vi "SUB-BLE Rx data Classify.vi"() -> (0 "data out":u8[](array[numeric]) format="%2x", 1 "Rx-set":bool=TRUE, 2 "Rx-mon":bool=TRUE)   [LabVIEW 2015]
doc: "Use this template to create an application that executes repeatedly until you click the Stop button. This template polls the state of the Stop button and does not use events. Use the Top-Level Application template (not available in the Base package) to create a single-loop application with event handling."
uses:
  Global 1.vi
panel:
  out "BLE Packet (buf)":u8[](array[numeric])
  out "BLE Packet (data)":u8[](array[numeric])
  out "BLE Packet":bool=TRUE
  # "BLE 수신 데이터를 분류: Monitoring/Setting data"
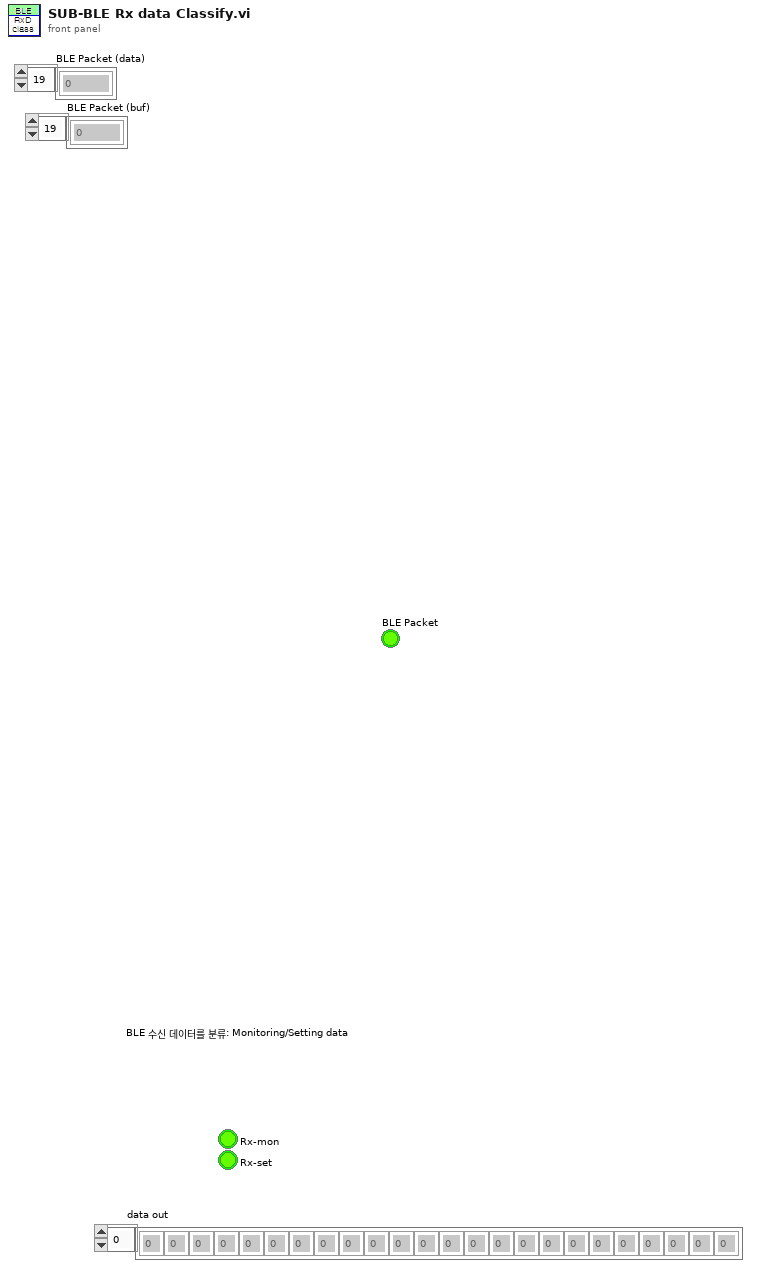
[diagram p1: front panel]
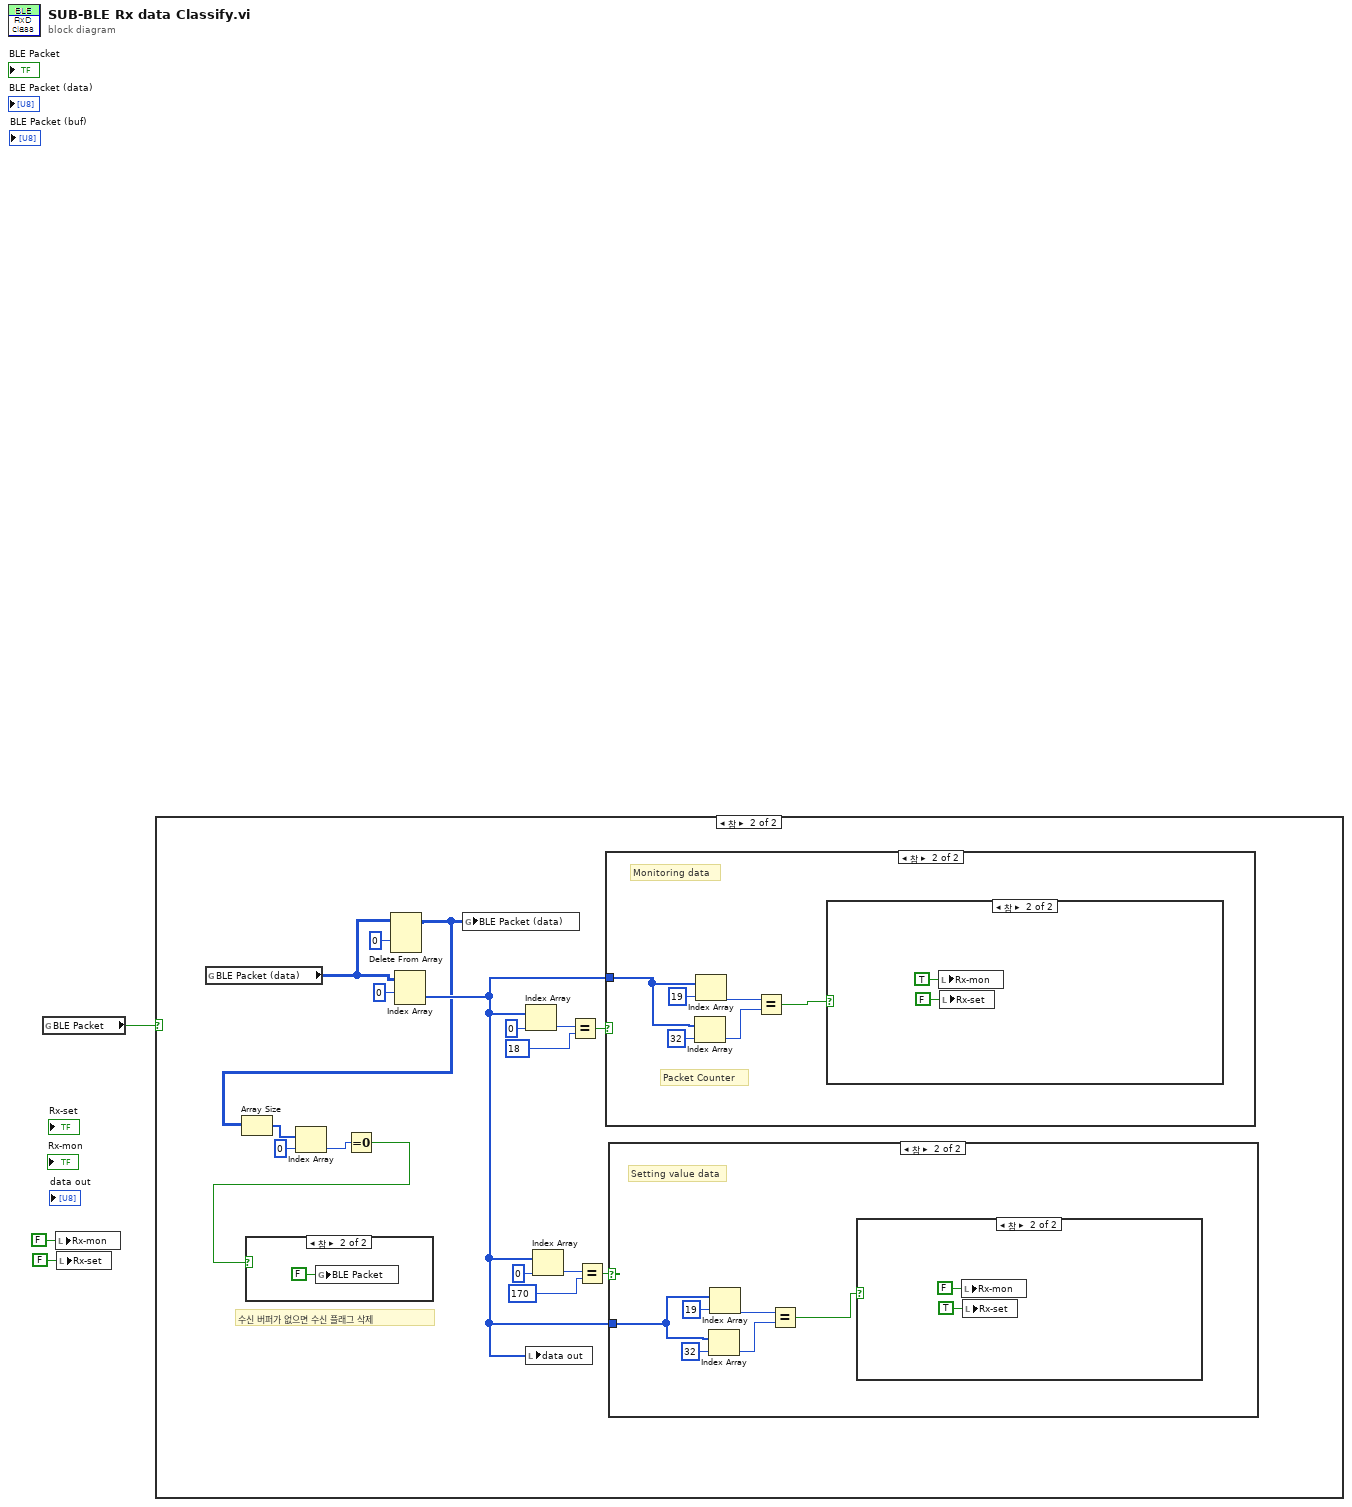
[diagram p0: block diagram]
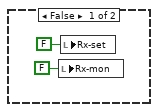
[diagram p2: hidden frame]
diagram:
  n1 = global read "Global 1.vi" "BLE Packet"() -> (w3:bool)
  n2 = local write "Rx-mon"(FALSE ("Rx-mon")) -> ()
  n3 = local write "Rx-set"(FALSE ("Rx-set")) -> ()
  n4 = case shown="참" w3 {
    frame False {
      n5 = local write "Rx-mon"(FALSE ("Rx-mon")) -> ()
      n6 = local write "Rx-set"(FALSE ("Rx-set")) -> ()
    }
    frame True {
      # "수신 버퍼가 없으면 수신 플래그 삭제"
      n7 = global read "Global 1.vi" "BLE Packet (data)"() -> (w12:u8[][])
      n8 = Delete From Array(array=w12, index (row)=0 ("인덱스 (행)")) -> (array with subset deleted=w10:u8[][])  [unwired: 2 in, 1 out]
      n9 = Array Size(array=w10) -> (size(s)=w9:i32[])
      n10 = Index Array(array=w9, index=0 ("인덱스")) -> (element=w7:i32)
      n11 = Equal To 0?(x=w7) -> (x = 0?=w6:bool)
      n12 = case shown="참" w6 {
        frame False {
        }
        frame True {
          n13 = global write "Global 1.vi" "BLE Packet"(FALSE ("BLE Packet")) -> ()
        }
      }
      n14 = Index Array(array=w12, index (row)=0 ("인덱스 (행)")) -> (element=w13:u8[])  [unwired: 1 in]
      n15 = global write "Global 1.vi" "BLE Packet (data)"(w10) -> ()
      n16 = Index Array(array=w13, index=0 ("인덱스")) -> (element=w21:u8)
      n17 = local write "data out"(w13) -> ()
      n18 = Index Array(array=w13, index=0 ("인덱스")) -> (element=w17:u8)
      n19 = Equal?(x=w21, y=18 ("인덱스")) -> (x = y?=w19:bool)
      n20 = Equal?(x=w17, y=170 ("인덱스")) -> (x = y?=w15:bool)
      n21 = case shown="참" w19 {
        tunnel: w13 -> [_ w33]
        frame False {
        }
        frame True {
          # "Monitoring data"
          # "Packet Counter"
          n22 = Index Array(array=w33, index=32 ("인덱스")) -> (element=w37:u8)
          n23 = Index Array(array=w33, index=19 ("인덱스")) -> (element=w36:u8)
          n24 = Equal?(x=w36, y=w37) -> (x = y?=w32:bool)
          n25 = case shown="참" w32 {
            frame False {
            }
            frame True {
              n26 = local write "Rx-mon"(TRUE ("Rx-mon")) -> ()
              n27 = local write "Rx-set"(FALSE ("Rx-set")) -> ()
            }
          }
        }
      }
      n28 = case shown="참" w15 {
        tunnel: w13 -> [_ w25]
        frame False {
        }
        frame True {
          # "Setting value data"
          n29 = Index Array(array=w25, index=32 ("인덱스")) -> (element=w26:u8)
          n30 = Index Array(array=w25, index=19 ("인덱스")) -> (element=w27:u8)
          n31 = Equal?(x=w27, y=w26) -> (x = y?=w24:bool)
          n32 = case shown="참" w24 {
            frame False {
            }
            frame True {
              n33 = local write "Rx-mon"(FALSE ("Rx-mon")) -> ()
              n34 = local write "Rx-set"(TRUE ("Rx-set")) -> ()
            }
          }
        }
      }
    }
  }
